vi "Adquisicio_projecte_InsEl (2).vi"() -> ()   [LabVIEW 2014]
uses:
  <vilib>/DAQmx/configure/timing.llb/DAQmx Timing (Sample Clock).vi
  <vilib>/DAQmx/read.llb/DAQmx Read (Analog 1D Wfm NChan NSamp).vi
panel:
  in  "Tab Control":enum32{"CH 1", "CH 2", "CH 3", "CH 4"}(tab)
  in  "T max 1":dbl
  in  "T min 1":dbl
  out "IND CH1":u32(colorbox)
  out "H CH1":dbl[](array[numeric])
  in  "T max  2":dbl
  in  "T min 2":dbl
  out "IND CH2":u32(colorbox)
  out "H CH2":dbl[](array[numeric])
  in  "T max 3":dbl
  in  "T min 3":dbl
  out "IND CH3":u32(colorbox)
  out "H CH3":dbl[](array[numeric])
  in  "T max 4":dbl
  in  "T min 4":dbl
  out "IND CH4":u32(colorbox)
  out "H CH4":dbl[](array[numeric])
  in  "PARAR PROGRAMA":bool
  out "?":bool
  out "?":bool
  out "?":bool
  out "?":bool
  out "MEDIA CH4":dbl
  out "MEDIA CH3":dbl
  out "MEDIA CH2":dbl
  out "MEDIA CH1":dbl
  out "Waveform Graph":waveform(dbl)[](graph)
  out "data":waveform(dbl)[](array[waveform])
  in  "Numero de Media":dbl
  in  "CH 4":bool
  in  "CH 3":bool
  in  "CH 2":bool
  in  "CH 1":bool
  in  "?":bool
  in  "Durada adquisició":dbl
  in  "Temps entre adquisicions":dbl
  in  "?":bool
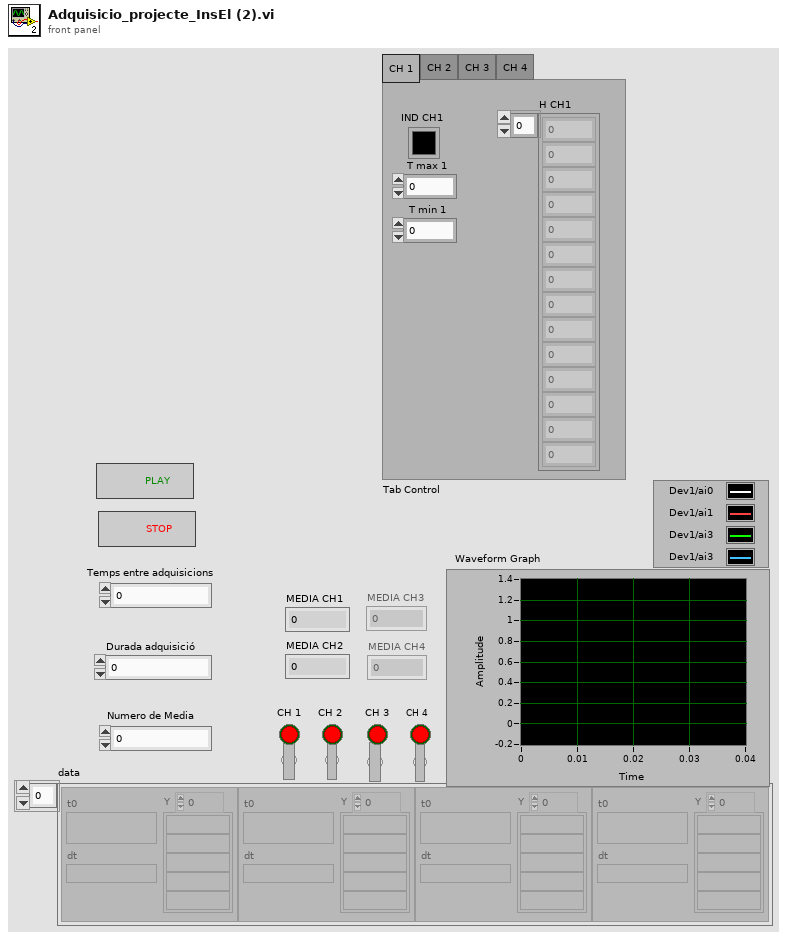
[diagram p1: front panel]
types:
  T1 = enum8{"Enabled", "Disabled", "Disabled and Grayed Out"}
  T2 = cluster{"CH 1":bool, "CH 2":bool, "CH 3":bool, "CH 4":bool}
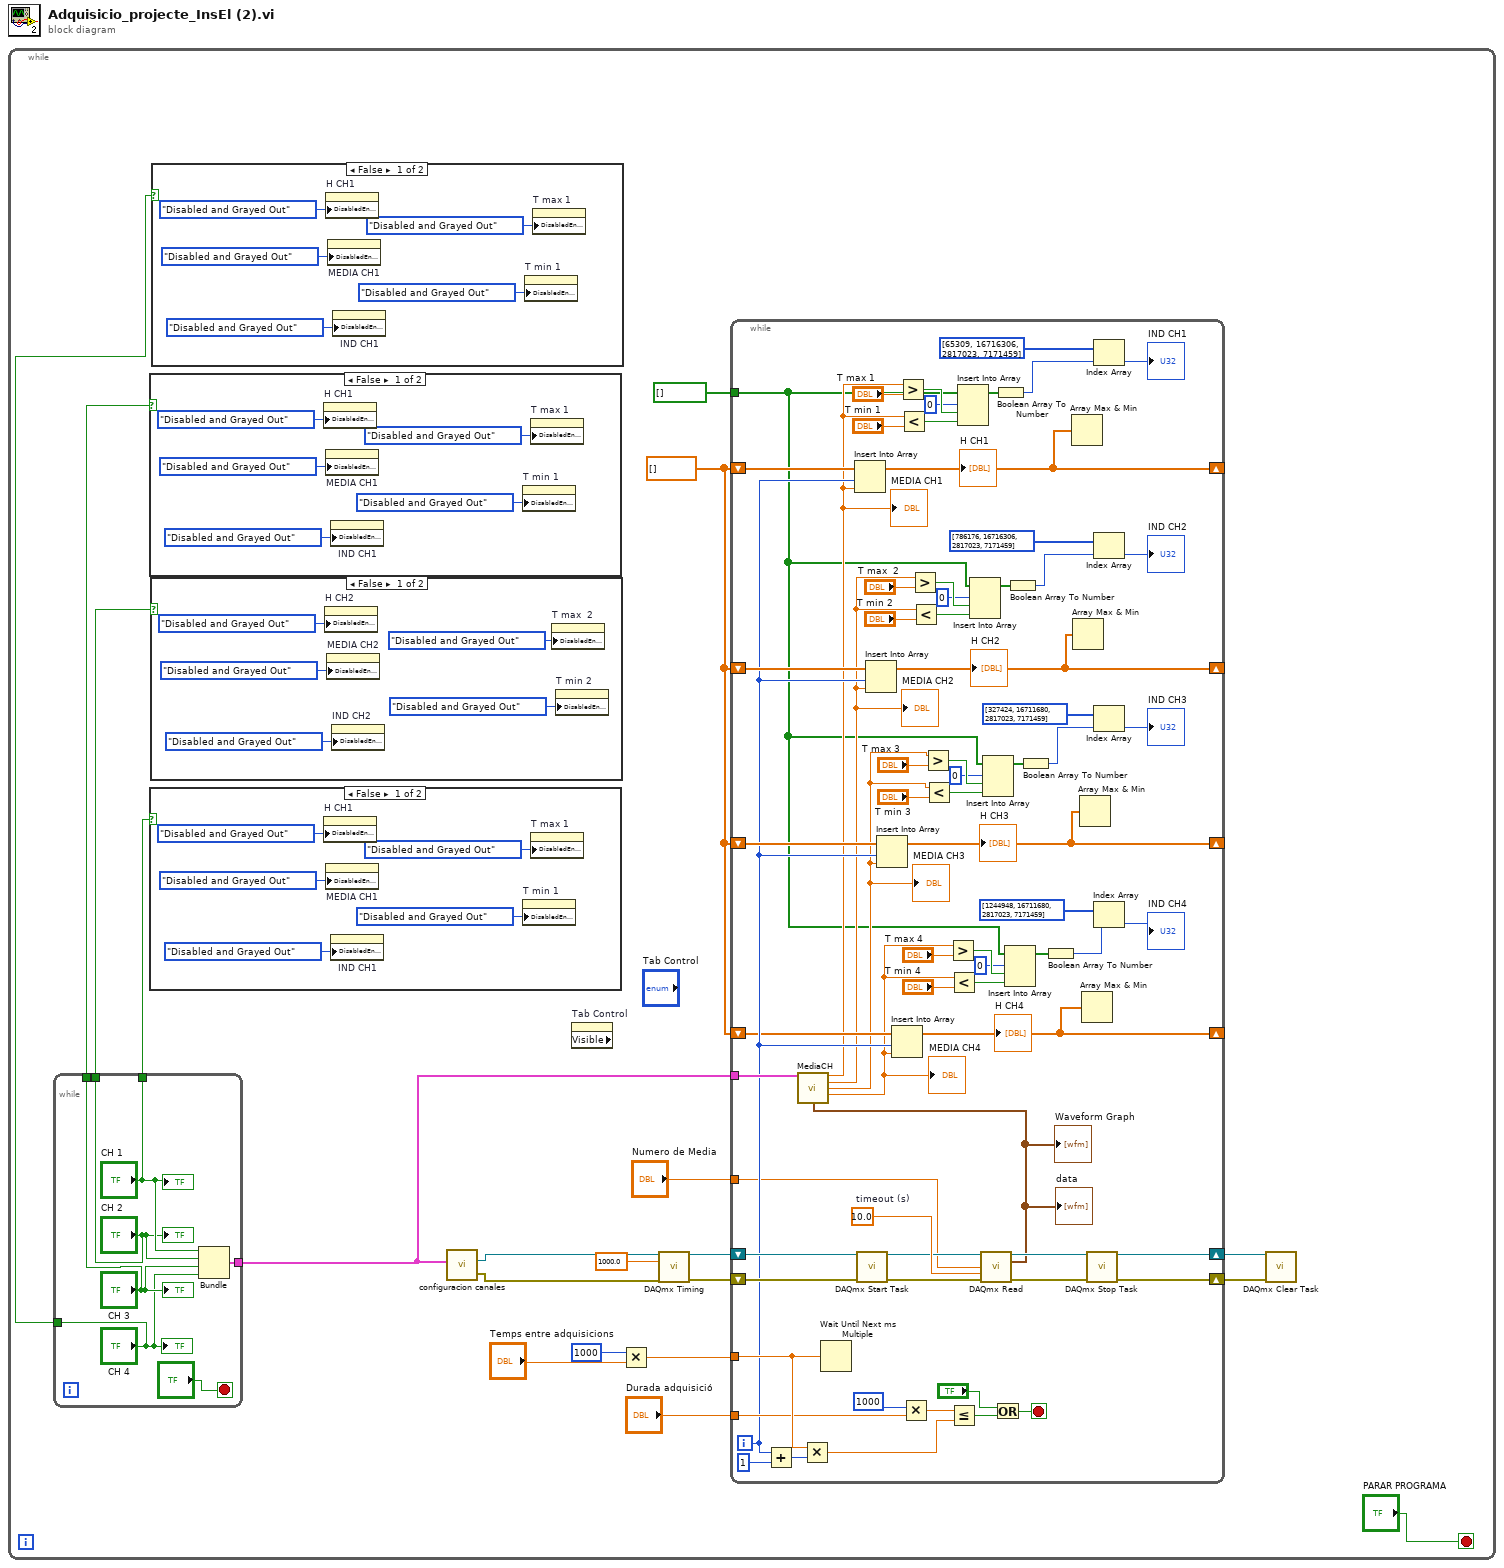
[diagram p0: block diagram]
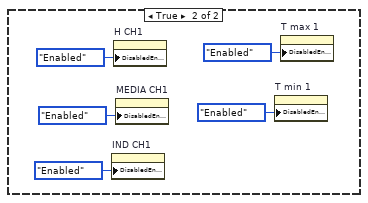
[diagram p2: hidden frame]
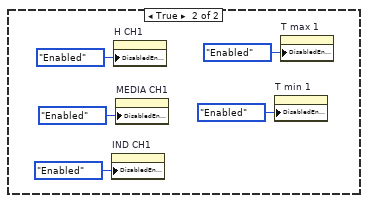
[diagram p3: hidden frame]
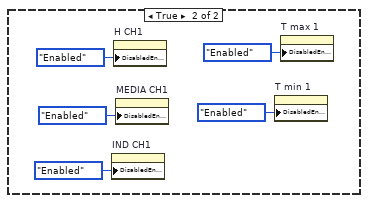
[diagram p4: hidden frame]
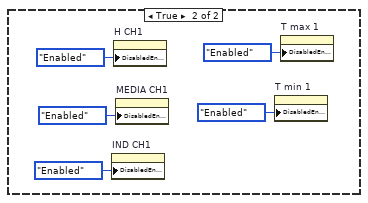
[diagram p5: hidden frame]
diagram:
  n1 = while {
    stop <- "PARAR PROGRAMA" stop-if-true
    w7 = dbl[] [] ("array")
    n2 = while {
      tunnel: [w66] -> w13
      tunnel: ["CH 1"] -> w4
      tunnel: ["CH 2"] -> w1
      tunnel: ["CH 3"] -> w2
      tunnel: ["CH 4"] -> w3
      stop <- "?" stop-if-true
      n3 = Bundle("CH 1"="CH 1", "CH 2"="CH 2", "CH 3"="CH 3", "CH 4"="CH 4") -> (w66:T2)  [unwired: 1 in]
      "?" <- "CH 1"
      "?" <- "CH 2"
      "?" <- "CH 3"
      "?" <- "CH 4"
    }
    n4 = case shown="False" w2 {
      frame False {
        n5 = property on="H CH1" class="Arr (strict)"("DisabledEnum"=T1."Disabled and Grayed Out" ("Disabled")) -> ()  [unwired: 2 in, 2 out]
        n6 = property on="MEDIA CH1" class="DigNum (strict)"("DisabledEnum"=T1."Disabled and Grayed Out" ("Disabled")) -> ()  [unwired: 2 in, 2 out]
        n7 = property on="IND CH1" class="ColBox"("DisabledEnum"=T1."Disabled and Grayed Out" ("Disabled")) -> ()  [unwired: 2 in, 2 out]
        n8 = property on="T min 1" class="DigNum (strict)"("DisabledEnum"=T1."Disabled and Grayed Out" ("Disabled")) -> ()  [unwired: 2 in, 2 out]
        n9 = property on="T max 1" class="DigNum (strict)"("DisabledEnum"=T1."Disabled and Grayed Out" ("Disabled")) -> ()  [unwired: 2 in, 2 out]
      }
      frame True {
        n10 = property on="IND CH1" class="ColBox"("DisabledEnum"=T1."Enabled" ("Disabled")) -> ()  [unwired: 2 in, 2 out]
        n11 = property on="H CH1" class="Arr (strict)"("DisabledEnum"=T1."Enabled" ("Disabled")) -> ()  [unwired: 2 in, 2 out]
        n12 = property on="MEDIA CH1" class="DigNum (strict)"("DisabledEnum"=T1."Enabled" ("Disabled")) -> ()  [unwired: 2 in, 2 out]
        n13 = property on="T min 1" class="DigNum (strict)"("DisabledEnum"=T1."Enabled" ("Disabled")) -> ()  [unwired: 2 in, 2 out]
        n14 = property on="T max 1" class="DigNum (strict)"("DisabledEnum"=T1."Enabled" ("Disabled")) -> ()  [unwired: 2 in, 2 out]
      }
    }
    n15 = case shown="False" w4 {
      frame False {
        n16 = property on="H CH1" class="Arr (strict)"("DisabledEnum"=T1."Disabled and Grayed Out" ("Disabled")) -> ()  [unwired: 2 in, 2 out]
        n17 = property on="MEDIA CH1" class="DigNum (strict)"("DisabledEnum"=T1."Disabled and Grayed Out" ("Disabled")) -> ()  [unwired: 2 in, 2 out]
        n18 = property on="IND CH1" class="ColBox"("DisabledEnum"=T1."Disabled and Grayed Out" ("Disabled")) -> ()  [unwired: 2 in, 2 out]
        n19 = property on="T min 1" class="DigNum (strict)"("DisabledEnum"=T1."Disabled and Grayed Out" ("Disabled")) -> ()  [unwired: 2 in, 2 out]
        n20 = property on="T max 1" class="DigNum (strict)"("DisabledEnum"=T1."Disabled and Grayed Out" ("Disabled")) -> ()  [unwired: 2 in, 2 out]
      }
      frame True {
        n21 = property on="IND CH1" class="ColBox"("DisabledEnum"=T1."Enabled" ("Disabled")) -> ()  [unwired: 2 in, 2 out]
        n22 = property on="H CH1" class="Arr (strict)"("DisabledEnum"=T1."Enabled" ("Disabled")) -> ()  [unwired: 2 in, 2 out]
        n23 = property on="MEDIA CH1" class="DigNum (strict)"("DisabledEnum"=T1."Enabled" ("Disabled")) -> ()  [unwired: 2 in, 2 out]
        n24 = property on="T min 1" class="DigNum (strict)"("DisabledEnum"=T1."Enabled" ("Disabled")) -> ()  [unwired: 2 in, 2 out]
        n25 = property on="T max 1" class="DigNum (strict)"("DisabledEnum"=T1."Enabled" ("Disabled")) -> ()  [unwired: 2 in, 2 out]
      }
    }
    n26 = case shown="False" w1 {
      frame False {
        n27 = property on="H CH2" class="Arr (strict)"("DisabledEnum"=T1."Disabled and Grayed Out" ("Disabled")) -> ()  [unwired: 2 in, 2 out]
        n28 = property on="MEDIA CH2" class="DigNum (strict)"("DisabledEnum"=T1."Disabled and Grayed Out" ("Disabled")) -> ()  [unwired: 2 in, 2 out]
        n29 = property on="IND CH2" class="ColBox"("DisabledEnum"=T1."Disabled and Grayed Out" ("Disabled")) -> ()  [unwired: 2 in, 2 out]
        n30 = property on="T max  2" class="DigNum (strict)"("DisabledEnum"=T1."Disabled and Grayed Out" ("Disabled")) -> ()  [unwired: 2 in, 2 out]
        n31 = property on="T min 2" class="DigNum (strict)"("DisabledEnum"=T1."Disabled and Grayed Out" ("Disabled")) -> ()  [unwired: 2 in, 2 out]
      }
      frame True {
        n32 = property on="IND CH1" class="ColBox"("DisabledEnum"=T1."Enabled" ("Disabled")) -> ()  [unwired: 2 in, 2 out]
        n33 = property on="H CH1" class="Arr (strict)"("DisabledEnum"=T1."Enabled" ("Disabled")) -> ()  [unwired: 2 in, 2 out]
        n34 = property on="MEDIA CH1" class="DigNum (strict)"("DisabledEnum"=T1."Enabled" ("Disabled")) -> ()  [unwired: 2 in, 2 out]
        n35 = property on="T min 1" class="DigNum (strict)"("DisabledEnum"=T1."Enabled" ("Disabled")) -> ()  [unwired: 2 in, 2 out]
        n36 = property on="T max 1" class="DigNum (strict)"("DisabledEnum"=T1."Enabled" ("Disabled")) -> ()  [unwired: 2 in, 2 out]
      }
    }
    n37 = case shown="False" w3 {
      frame False {
        n38 = property on="H CH1" class="Arr (strict)"("DisabledEnum"=T1."Disabled and Grayed Out" ("Disabled")) -> ()  [unwired: 2 in, 2 out]
        n39 = property on="MEDIA CH1" class="DigNum (strict)"("DisabledEnum"=T1."Disabled and Grayed Out" ("Disabled")) -> ()  [unwired: 2 in, 2 out]
        n40 = property on="IND CH1" class="ColBox"("DisabledEnum"=T1."Disabled and Grayed Out" ("Disabled")) -> ()  [unwired: 2 in, 2 out]
        n41 = property on="T min 1" class="DigNum (strict)"("DisabledEnum"=T1."Disabled and Grayed Out" ("Disabled")) -> ()  [unwired: 2 in, 2 out]
        n42 = property on="T max 1" class="DigNum (strict)"("DisabledEnum"=T1."Disabled and Grayed Out" ("Disabled")) -> ()  [unwired: 2 in, 2 out]
      }
      frame True {
        n43 = property on="IND CH1" class="ColBox"("DisabledEnum"=T1."Enabled" ("Disabled")) -> ()  [unwired: 2 in, 2 out]
        n44 = property on="H CH1" class="Arr (strict)"("DisabledEnum"=T1."Enabled" ("Disabled")) -> ()  [unwired: 2 in, 2 out]
        n45 = property on="MEDIA CH1" class="DigNum (strict)"("DisabledEnum"=T1."Enabled" ("Disabled")) -> ()  [unwired: 2 in, 2 out]
        n46 = property on="T min 1" class="DigNum (strict)"("DisabledEnum"=T1."Enabled" ("Disabled")) -> ()  [unwired: 2 in, 2 out]
        n47 = property on="T max 1" class="DigNum (strict)"("DisabledEnum"=T1."Enabled" ("Disabled")) -> ()  [unwired: 2 in, 2 out]
      }
    }
    n48 = call "configuracion canales.vi"("input cluster"=w13) -> ("error out"=w14:errorcluster, "task out"=w15:refnum<k21>)  [unwired: 3 in]
    n49 = property on="Tab Control" class="TabCtl (strict)" props=["Visible"]() -> ()  [unwired: 2 in, 3 out]
    n50 = Multiply(x=1000, y="Temps entre adquisicions") -> (x*y=w10:dbl)
    n51 = call-poly <vilib>:"DAQmx Timing.vi"("task/channels in"=w15, "rate"=1000.0, "error in"=w14) -> ("task out"=w18:refnum<k21>, "error out"=w17:errorcluster)  [unwired: 11 in]
    n52 = while {
      shift-right: [w135] -> w20
      shift-left: w18 -> [w131]
      shift-right: [w134] -> w19
      shift-left: w17 -> [w120]
      tunnel: w10 -> [w125]
      tunnel: w13 -> [w124]
      tunnel: "Numero de Media" -> [w67]
      tunnel: "Durada adquisició" -> [w121]
      shift-right: [w69] -> _
      shift-left: w7 -> [w117]
      shift-right: [w70] -> _
      shift-left: w7 -> [w116]
      shift-right: [w68] -> _
      shift-left: w7 -> [w115]
      shift-right: [w71] -> _
      shift-left: w7 -> [w113]
      tunnel: bool[] [] ("array") -> [w77]
      i -> [w114]
      stop <- w122 stop-if-true
      w138 = 10.0  # timeout (s)
      n53 = Add(x=w114, y=1 ("x")) -> (x+y=w123:i32)
      n54 = Multiply(x=w125, y=w123) -> (x*y=w126:dbl)
      n55 = Wait Until Next ms Multiple(millisecond multiple=w125) -> ()  [unwired: 1 out]
      n56 = call <vilib>:"DAQmx Start Task.vi"("task/channels in"=w131, "error in"=w120) -> ("task out"=w136:refnum<k21>, "error out"=w137:errorcluster)  [unwired: 12 in]
      n57 = Multiply(x=1000, y=w121) -> (x*y=w128:dbl)
      n58 = Less Or Equal?(x=w128, y=w126) -> (x <= y?=w127:bool)
      n59 = call-poly <vilib>:"DAQmx Read.vi"("task/channels in"=w136, "number of samples per channel"=w67, "timeout"=w138, "error in"=w137) -> ("task out"=w133:refnum<k21>, "data"=w118:waveform(dbl)[], "error out"=w132:errorcluster)  [unwired: 9 in]
      "data" <- w118
      "Waveform Graph" <- w118
      n60 = call "MediaCH.vi"("input cluster"=w124, "Data"=w118) -> ("Mitja CH1"=w111:dbl, "Mitja CH2"=w95:dbl, "Mitja CH3"=w86:dbl, "Mitja CH4"=w76:dbl)  [unwired: 10 in]
      "MEDIA CH3" <- w86
      "MEDIA CH4" <- w76
      "MEDIA CH1" <- w111
      "MEDIA CH2" <- w95
      n61 = Insert Into Array(array=w117, index=w114, new element=w111) -> (w69:dbl[])
      "H CH1" <- w69
      n62 = Insert Into Array(array=w116, index=w114, new element=w95) -> (w70:dbl[])
      "H CH2" <- w70
      n63 = Insert Into Array(array=w115, index=w114, new element=w86) -> (w68:dbl[])
      "H CH3" <- w68
      n64 = Insert Into Array(array=w113, index=w114, new element=w76) -> (w71:dbl[])
      "H CH4" <- w71
      n65 = Greater?(x=w111, y="T max 1") -> (0:w109:bool)
      n66 = Less?(x=w111, y="T min 1") -> (x < y?=w108:bool)
      n67 = Greater?(x=w95, y="T max  2") -> (0:w101:bool)
      n68 = Less?(x=w95, y="T min 2") -> (x < y?=w100:bool)
      n69 = Greater?(x=w86, y="T max 3") -> (0:w93:bool)
      n70 = Less?(x=w86, y="T min 3") -> (x < y?=w92:bool)
      n71 = Greater?(x=w76, y="T max 4") -> (0:w84:bool)
      n72 = Less?(x=w76, y="T min 4") -> (x < y?=w83:bool)
      n73 = Insert Into Array(array=w77, index=0, new element #1=w109, new element #2=w108) -> (w106:bool[])
      n74 = Insert Into Array(array=w77, index=0, new element #1=w101, new element #2=w100) -> (w98:bool[])
      n75 = Insert Into Array(array=w77, index=0, new element #1=w93, new element #2=w92) -> (w90:bool[])
      n76 = Or(x="?", y=w127) -> (x .or. y?=w122:bool)
      n77 = Boolean Array To Number(Boolean array=w106) -> (number=w104:u32)
      n78 = Insert Into Array(array=w77, index=0, new element #1=w84, new element #2=w83) -> (w81:bool[])
      n79 = Boolean Array To Number(Boolean array=w98) -> (number=w96:u32)
      n80 = Boolean Array To Number(Boolean array=w90) -> (number=w88:u32)
      n81 = Boolean Array To Number(Boolean array=w81) -> (number=w78:u32)
      n82 = Array Max & Min(array=w69) -> ()  [unwired: 4 out]
      n83 = Array Max & Min(array=w70) -> ()  [unwired: 4 out]
      n84 = Array Max & Min(array=w68) -> ()  [unwired: 4 out]
      n85 = Array Max & Min(array=w71) -> ()  [unwired: 4 out]
      n86 = call <vilib>:"DAQmx Stop Task.vi"("task/channels in"=w133, "error in"=w132) -> ("task out"=w135:refnum<k21>, "error out"=w134:errorcluster)  [unwired: 12 in]
      n87 = Index Array(array=u32[] [65309, 16716306, 2817023, 7171459], index=w104) -> (element=→"IND CH1":u32)
      n88 = Index Array(array=u32[] [786176, 16716306, 2817023, 7171459], index=w96) -> (element=→"IND CH2":u32)
      n89 = Index Array(array=u32[] [327424, 16711680, 2817023, 7171459], index=w88) -> (element=→"IND CH3":u32)
      n90 = Index Array(array=u32[] [1244948, 16711680, 2817023, 7171459], index=w78) -> (element=→"IND CH4":u32)
    }
    n91 = call <vilib>:"DAQmx Clear Task.vi"("task in"=w20, "error in"=w19) -> ()  [unwired: 13 in, 1 out]
  }
